vi "InsertDataFlowStep.vi"(7 "type":T1, 8 "error in (no error)":errorcluster, 9 "add to beginning":bool, 10 "previous data flow step":string, 11 "new data flow step":string) -> (0 "error out":errorcluster)   [LabVIEW 2017, in "DataFlow.lvlib"]
doc: "Adds a process to a specific position within the Dataflow Script."
uses:
  <vilib>/addons/InsightCM/Devices/Shared/Common/DataFlow/DataFlow.lvlib
  <vilib>/addons/InsightCM/Devices/Shared/Common/DataFlow/controls/Type.ctl
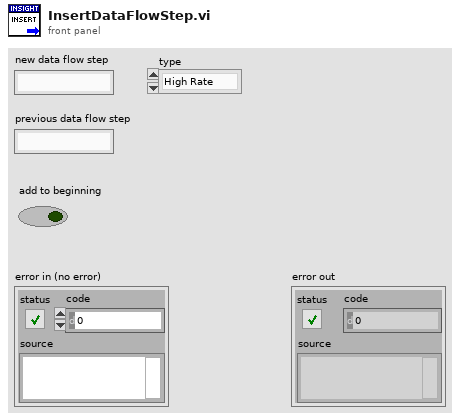
[diagram p1: front panel]
types:
  T1 = typedef "DataFlow.lvlib/Type.ctl" = enum16{"High Rate", "Low Rate", "Burst Mode"}
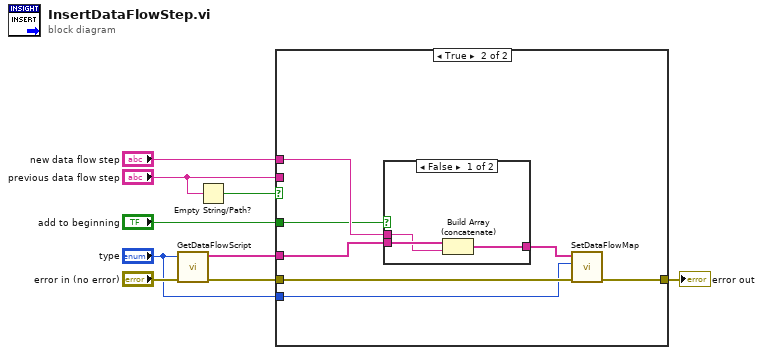
[diagram p0: block diagram]
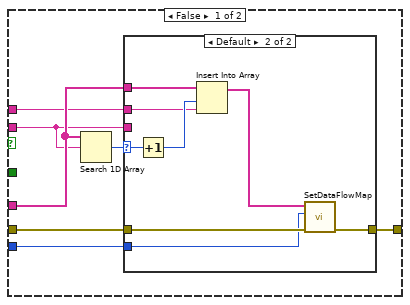
[diagram p2: hidden frame]
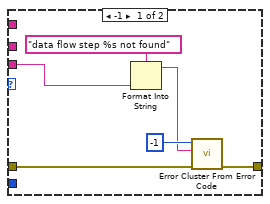
[diagram p3: hidden frame]
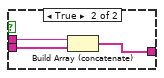
[diagram p4: hidden frame]
diagram:
  n1 = call <vilib>:"GetDataFlowScript.vi"("error in (no error)"="error in (no error)", "type"="type") -> ("error out"=w8:errorcluster, "Dataflow script"=w7:string[])  [unwired: 7 in, 1 out]
  n2 = Empty String/Path?(string/path="previous data flow step") -> (empty?=w3:bool)
  n3 = case shown="True" w3 {
    tunnel: w8 -> [w15 w37]
    tunnel: w7 -> [w14 w35]
    tunnel: [w13 w36] -> w6
    tunnel: "new data flow step" -> [w12 w34]
    tunnel: "previous data flow step" -> [w11 _]
    tunnel: "add to beginning" -> [_ w32]
    tunnel: "type" -> [w10 w31]
    frame False {
      n4 = Search 1D Array(1D array=w14, element=w11) -> (index of element=w16:i32)  [unwired: 1 in]
      n5 = case shown="Default" w16 {
        selector: w16 -> [_ w27]
        tunnel: w14 -> [_ w30]
        tunnel: w12 -> [_ w28]
        tunnel: w15 -> [w22 w26]
        tunnel: [w21 w25] -> w13
        tunnel: w11 -> [w19 _]
        tunnel: w10 -> [_ w23]
        frame -1 {
          n6 = Format Into String(format string="data flow step %s not found", w19) -> (resulting string=w18:string)  [unwired: 2 in, 1 out]
          n7 = call <vilib>:"Error Cluster From Error Code.vi"("error in (no error)"=w22, "error message (\"\")"=w18, "error code (0)"=-1) -> ("error out"=w21:errorcluster)  [unwired: 6 in]
        }
        frame Default {
          n8 = Increment(x=w27) -> (x+1=w29:i32)
          n9 = Insert Into Array(array=w30, index=w29, new element=w28) -> (w24:string[])
          n10 = call <vilib>:"SetDataFlowMap.vi"("error in (no error)"=w26, "type"=w23, "Dataflow script"=w24) -> ("error out"=w25:errorcluster)  [unwired: 8 in]
        }
      }
    }
    frame True {
      n11 = case shown="False" w32 {
        tunnel: w35 -> [w40 w43]
        tunnel: w34 -> [w39 w42]
        tunnel: [w38 w41] -> w33
        frame False {
          n12 = Build Array (concatenate)(w40, w39) -> (w38:string[])
        }
        frame True {
          n13 = Build Array (concatenate)(w42, w43) -> (w41:string[])
        }
      }
      n14 = call <vilib>:"SetDataFlowMap.vi"("error in (no error)"=w37, "type"=w31, "Dataflow script"=w33) -> ("error out"=w36:errorcluster)  [unwired: 8 in]
    }
  }
  "error out" <- w6
